vi "Disconnect From Network.vi"(8 "error in (no error)":errorcluster, 11 "ESP8266 in":refnum<class "ESP8266.lvclass">) -> (0 "error out":errorcluster, 3 "ESP8266 out":refnum<class "ESP8266.lvclass">)   [LabVIEW 2020, in "ESP8266.lvclass"]
uses:
  ESP8266.lvclass
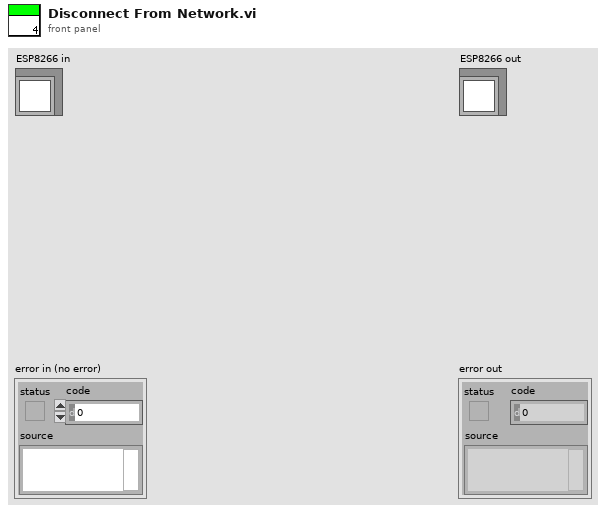
[diagram p1: front panel]
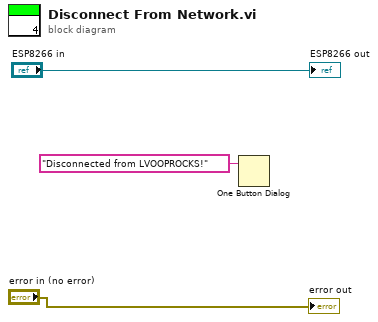
[diagram p0: block diagram]
diagram:
  n1 = One Button Dialog(message="Disconnected from LVOOPROCKS!") -> ()  [unwired: 1 in, 1 out]
  "error out" <- "error in (no error)"
  "ESP8266 out" <- "ESP8266 in"
